vi "CLSUIP_Populate Virtual Folder Names.vi"(6 "error out in":errorcluster, 8 "Place new accessors in this folder \n(select existing or type name for new folder):":refnum<vi>, 9 "DNL_LVClassLibrary Refnum":refnum<vi>) -> (0 "error out":errorcluster)   [LabVIEW 2021, in "MemberVICreation.lvlib"]
uses:
  <resource>/Framework/Providers/LVClassLibrary/NewAccessors/MemberVICreation.lvlib
panel:
  in  "Initial Text for \"No Folder\"":string[](array[string])=["--- No Folder ---"]
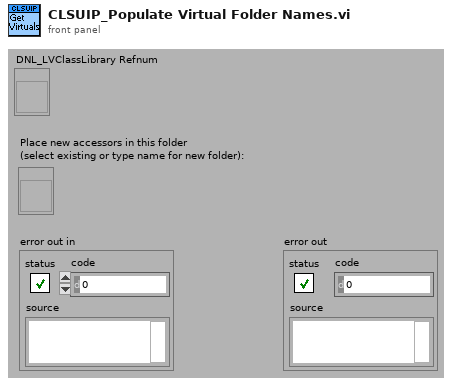
[diagram p1: front panel]
types:
  T1 = typedef "LIBUIP_item_type.ctl" = enum16{"None", "ParentLib", "Property Def Item", "VI", "Non-VI", "Folder", "Library", "Menu", "XI Ability VI", "XI Method VI", "XI Property VI", "Property Folder", "Class Private Data"}
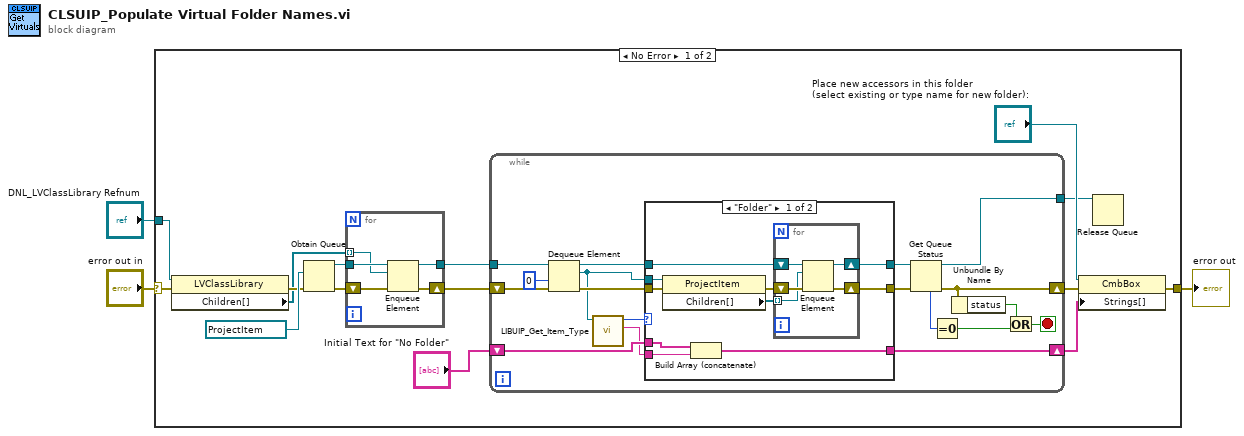
[diagram p0: block diagram]
diagram:
  n1 = case shown="No Error" "error out in" {
    selector: "error out in" -> [w14 w60]
    tunnel: [w13 w60] -> w2
    tunnel: "DNL_LVClassLibrary Refnum" -> [w18 _]
    frame No Error {
      n2 = property class="LVClassLibrary"(reference=w18, error in=w14) -> (error out=w11:errorcluster, "Children[]"=w6:refnum<vi>[])  [unwired: 1 out]
      n3 = Obtain Queue(element data type=refnum<vi> refnum ("ProjectItem Refnum"), error in (no error)=w11) -> (queue out=w10:refnum<queue>, error out=w9:errorcluster)  [unwired: 2 in, 2 out]
      n4 = for {
        tunnel: w10 -> [w59]
        shift-right: [w57] -> w7
        shift-left: w9 -> [w58]
        tunnel: [w56] -> w8
        tunnel: w6 -> [w55] mode=indexing
        n5 = Enqueue Element(queue=w59, element=w55, error in (no error)=w58) -> (queue out=w56:refnum<queue>, error out=w57:errorcluster)  [unwired: 2 out]
      }
      n6 = while {
        shift-right: [w34] -> w15
        shift-left: "Initial Text for \"No Folder\"" -> [w35]
        tunnel: w8 -> [w31]
        shift-right: [w20] -> w5
        shift-left: w7 -> [w32]
        tunnel: [w22] -> w4
        stop <- w21 stop-if-true
        n7 = Dequeue Element(queue=w31, timeout in ms (-1)=0, error in (no error)=w32) -> (queue out=w28:refnum<queue>, element=w29:refnum<vi>, error out=w30:errorcluster)  [unwired: 1 out]
        n8 = call <resource>:"LIBUIP_Get_Item_Type.vi"("ProjectItem Refnum"=w29) -> ("Name"=w33:string, "Type"=w36:T1)  [unwired: 1 in, 8 out]
        n9 = case shown="\"Folder\"" w36 {
          tunnel: w35 -> [w46 w54]
          tunnel: [w45 w54] -> w34
          tunnel: w33 -> [w44 _]
          tunnel: w30 -> [w43 w53]
          tunnel: w29 -> [w42 _]
          tunnel: [w41 w53] -> w26
          tunnel: w28 -> [w39 w52]
          tunnel: [w37 w52] -> w25
          frame "Folder" {
            n10 = property class="ProjectItem"(reference=w42, error in=w43) -> (error out=w40:errorcluster, "Children[]"=w38:refnum<vi>[])  [unwired: 1 out]
            n11 = Build Array (concatenate)(w46, w44) -> (w45:string[])
            n12 = for {
              shift-right: [w51] -> w41
              shift-left: w40 -> [w50]
              tunnel: w38 -> [w48] mode=indexing
              shift-right: [w47] -> w37
              shift-left: w39 -> [w49]
              n13 = Enqueue Element(queue=w49, element=w48, error in (no error)=w50) -> (queue out=w47:refnum<queue>, error out=w51:errorcluster)  [unwired: 2 out]
            }
          }
          frame Default {
          }
        }
        n14 = Get Queue Status(queue=w25, error in (no error)=w26) -> (queue out=w22:refnum<queue>, error out=w20:errorcluster, # elements in queue=w24:i32)  [unwired: 6 out]
        n15 = Equal To 0?(x=w24) -> (x = 0?=w23:bool)
        n16 = Unbundle By Name(w20) -> ("status"=w19:bool)
        n17 = Or(x=w19, y=w23) -> (x .or. y?=w21:bool)
      }
      n18 = property class="CmbBox"(reference="Place new accessors in this folder \n(select existing or type name for new folder):", error in=w5, "Strings[]"=w15) -> (error out=w13:errorcluster)  [unwired: 1 out]
      n19 = Release Queue(queue=w4) -> ()  [unwired: 1 in, 4 out]
    }
    frame Error {
    }
  }
  "error out" <- w2
